vi "Model--Create New Group.vi"(8 "error in":errorcluster, 11 "Selector in":refnum<class "Selector.lvclass">) -> (0 "error out":errorcluster, 1 "Group":string, 2 "Name":string, 3 "Selector out":refnum<class "Selector.lvclass">)   [LabVIEW 2019, in "Selector.lvclass"]
uses:
  Selector.lvclass
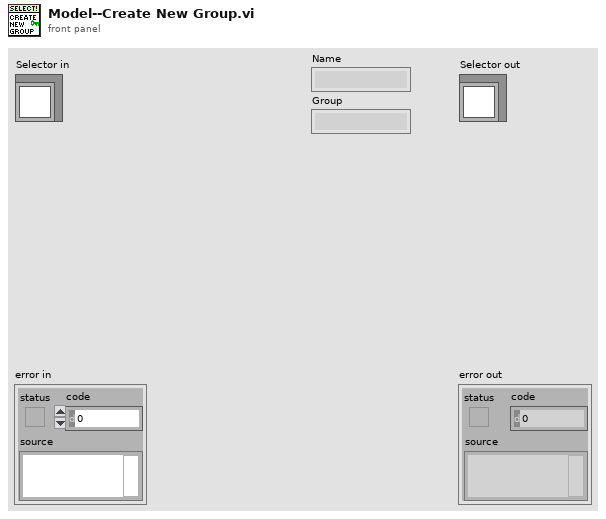
[diagram p1: front panel]
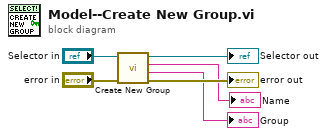
[diagram p0: block diagram]
diagram:
  n1 = call-dynamic "Create New Group.vi"("error in (no error)"="error in", "Selector in"="Selector in") -> ("error out"=→"error out":errorcluster, "Group"=→"Group":string, "Name"=→"Name":string, "Selector out"=→"Selector out":refnum<class "Selector.lvclass">)  [unwired: 6 in]
